vi "Lookup Channel Index.vi"(8 "error in (no error)":errorcluster, 10 "Channel Name":string, 11 "GroupAbstract in":refnum<class "Group.lvclass">) -> (0 "error out":errorcluster, 2 "Index":i32, 3 "GroupAbstract out":refnum<class "Group.lvclass">)   [LabVIEW 2020, in "Vecto.lvlib" / "Group.lvclass"]
uses:
  Group.lvclass
  Group.lvclass/Group.ctl
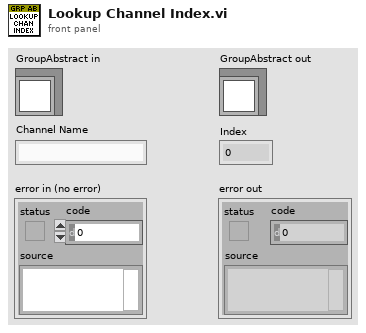
[diagram p1: front panel]
types:
  T1 = typedef "Vecto.lvlib/GroupAbstract.lvclass/Ref.ctl" = cluster{"Channel Index Map":map{string, i32}, "Channel Info":T2[]}
  T2 = typedef "Vecto.lvlib/Channel Info.ctl" = cluster{"Name":string, "Group":string, "Owning Node":string, "Owning Task":string, "Resource":string}
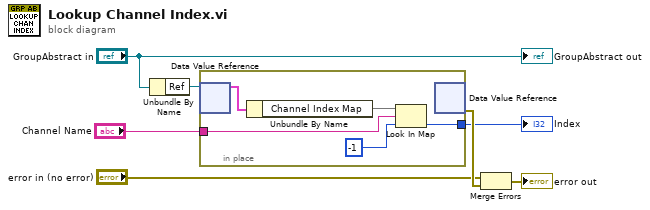
[diagram p0: block diagram]
diagram:
  n1 = Unbundle By Name("GroupAbstract in") -> ("Ref"=w7:refnum<data-value>)
  n2 = in-place {
    in-place-border: "Channel Name" -> [w10]
    in-place-border: [w9] -> w3
    n3 = in-place-dvr #1(w7) -> (w12:T1)  [unwired: 1 out]
    n4 = Unbundle By Name(w12) -> ("Channel Index Map"=w11:map{string, i32})
    n5 = Look In Map(map=w11, key=w10, default value=-1) -> (value=w9:i32)  [unwired: 1 out]
    n6 = in-place-dvr #1() -> (w6:errorcluster)  [unwired: 1 in, 1 out]
  }
  "Index" <- w3
  n7 = Merge Errors("error in (no error)", w6) -> (→"error out":errorcluster)
  "GroupAbstract out" <- "GroupAbstract in"
